vi "ConfigUtilities - Get Tx Packet Information.vi"(8 "error in (no error)":errorcluster, 11 "Custom Device Ref in":T1 format="%.0x") -> (0 "error out":errorcluster, 1 "Tx Ref Array":T2(array[cluster]) {"VS Refs" format="%.0x"}, 2 "Tx Packet Info Array":T3[](array[typedef]) {"Endianness" items=["big-endian"=0, "little-indian"=2]}, 3 "Custom Device Ref out":T1 format="%.0x")   [LabVIEW 2016, in "UDP-Custom-Device System Explorer.lvlib"]
uses:
  UDP-Custom-Device System Explorer.lvlib
  Shared/Tx.PacketInfo.ctl
  Types/Channel Data Type.ctl
  Shared/Header Details.ctl
  <vilib>/NI Veristand/Custom Device API/Custom Device Item Ref.ctl
  Shared/Constants.vi
  <vilib>/NI Veristand/Custom Device API/Get Item Property (I32).vi
  <vilib>/NI Veristand/Custom Device API/Get Item Property (String).vi
  <vilib>/NI Veristand/Custom Device API/Get Item Property (U16).vi
  <vilib>/NI Veristand/Custom Device API/Get Item Property (Boolean).vi
  <vilib>/NI Veristand/Custom Device API/Get Item Property (U32).vi
  Shared/UDP-Custom-Device Shared.lvlib
  <vilib>/NI VeriStand/Custom Device API/Custom Device API.lvlib
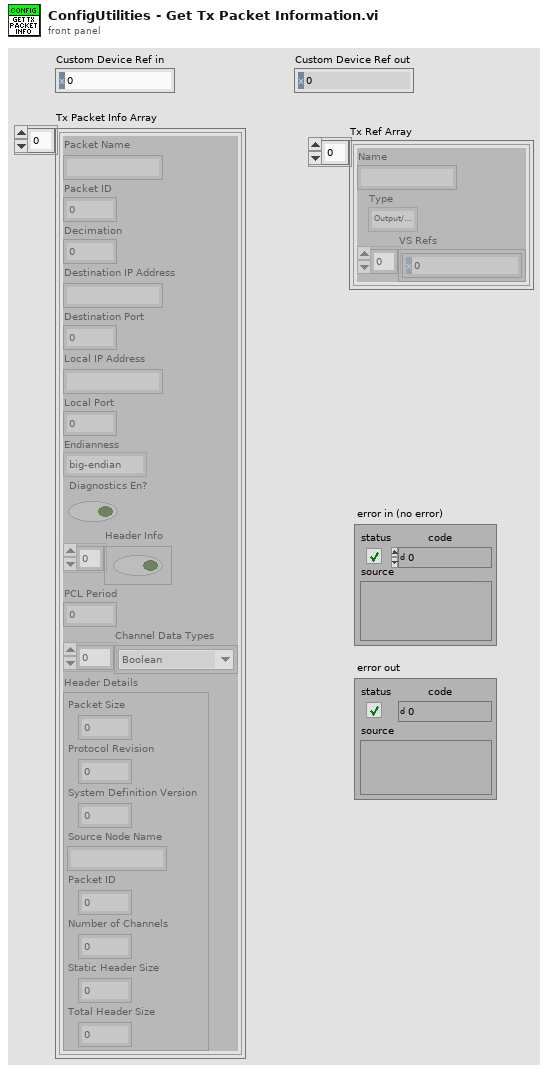
[diagram p1: front panel]
types:
  T1 = typedef "Custom Device API.lvlib/Custom Device Item Ref.ctl" = u64
  T2 = cluster{"Name":string, "Type":enum16{"Output/Write", "Input/Read", "Input/ReadWrite"}, "VS Refs":T1[]}[]
  T3 = typedef "UDP-Custom-Device Shared.lvlib/Tx.PacketInfo.ctl" = cluster{"Packet Name":string, "Packet ID":i32, "Decimation":u16, "Destination IP Address":string, "Destination Port":i32, "Local IP Address":string, "Local Port":i32, "Endianness":u16, "Diagnostics En?":bool, "Header Info":bool[], "PCL Period":u32, "Channel Data Types":T4[], "Header Details":T5}
  T4 = typedef "UDP-Custom-Device Shared.lvlib/Channel Data Type.ctl" = enum16{"Boolean", "Single", "Double", "I8", "I16", "I32", "I64", "U8", "U16", "U32", "U64"}
  T5 = typedef "UDP-Custom-Device Shared.lvlib/Header Details.ctl" = cluster{"Packet Size":u16, "Protocol Revision":u8, "System Definition Version":u64, "Source Node Name":string, "Packet ID":u32, "Number of Channels":u32, "Static Header Size":u16, "Total Header Size":u16}
  T6 = cluster{"Name":string, "Type":enum16{"Output/Write", "Input/Read", "Input/ReadWrite"}, "VS Refs":T1[]}
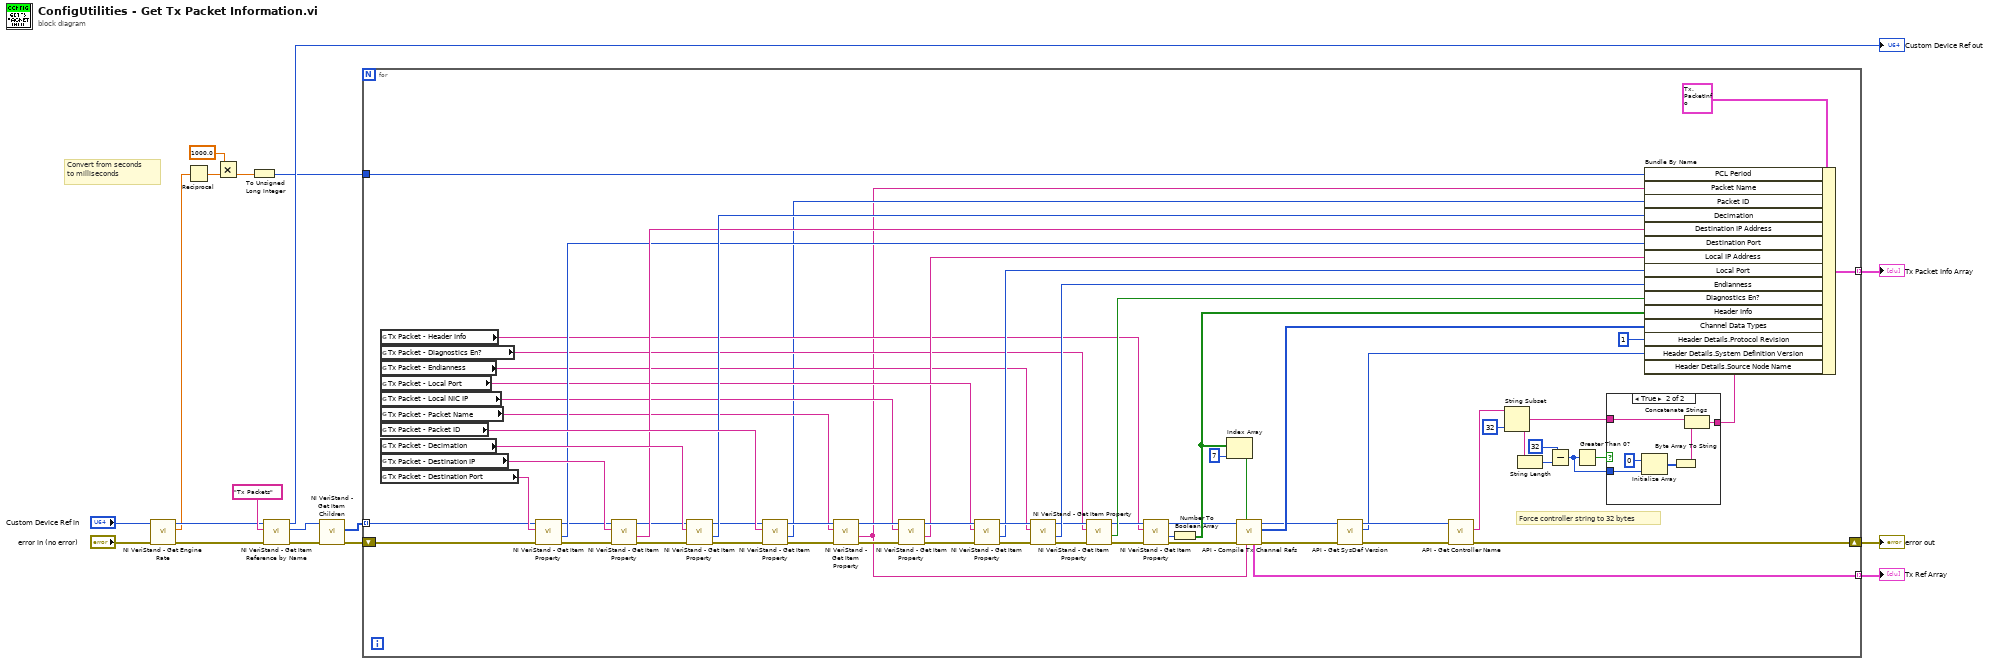
[diagram p0: block diagram]
diagram:
  # "Convert from seconds\nto milliseconds"
  n1 = call <vilib>:"NI VeriStand - Get Engine Rate.vi"("error in (no error)"="error in (no error)", "Item Ref in"="Custom Device Ref in") -> ("error out"=w7:errorcluster, "Rate (Hz)"=w5:dbl, "Item Ref out"=w6:T1)  [unwired: 7 in]
  n2 = Reciprocal(x=w5) -> (1/x=w1:dbl)
  n3 = Multiply(x=1000.0, y=w1) -> (x*y=w3:dbl)
  n4 = To Unsigned Long Integer(number=w3) -> (unsigned 32bit integer=w4:u32)
  n5 = call <vilib>:"NI VeriStand - Get Item Reference by Name.vi"("error in (no error)"=w7, "Item Name"="Tx Packets", "Parent Ref in"=w6) -> ("error out"=w13:errorcluster, "Item Ref"=w11:T1, "Parent Ref out"=→"Custom Device Ref out":T1)  [unwired: 5 in, 1 out]
  n6 = call <vilib>:"NI VeriStand - Get Item Children.vi"("error in (no error)"=w13, "Item Ref in"=w11) -> ("error out"=w16:errorcluster, "Child Refs"=w15:T1[])  [unwired: 6 in, 2 out]
  n7 = for {
    shift-right: [w32] -> w18
    shift-left: w16 -> [w83]
    tunnel: [w66] -> w17 mode=indexing
    tunnel: w15 -> [w65] mode=indexing
    tunnel: [w35] -> w14 mode=indexing
    tunnel: w4 -> [w44]
    # "Force controller string to 32 bytes"
    n8 = global read "Constants.vi" "Tx Packet - Header Info"() -> (w46:string)
    n9 = global read "Constants.vi" "Tx Packet - Diagnostics En?"() -> (w48:string)
    n10 = global read "Constants.vi" "Tx Packet - Endianness"() -> (w52:string)
    n11 = global read "Constants.vi" "Tx Packet - Local Port"() -> (w59:string)
    n12 = global read "Constants.vi" "Tx Packet - Local NIC IP"() -> (w60:string)
    n13 = global read "Constants.vi" "Tx Packet - Packet Name"() -> (w43:string)
    n14 = global read "Constants.vi" "Tx Packet - Packet ID"() -> (w79:string)
    n15 = global read "Constants.vi" "Tx Packet - Decimation"() -> (w80:string)
    n16 = global read "Constants.vi" "Tx Packet - Destination IP"() -> (w81:string)
    n17 = global read "Constants.vi" "Tx Packet - Destination Port"() -> (w82:string)
    n18 = call-poly <vilib>:"NI VeriStand - Get Item Property.vi"("error in (no error)"=w83, "Property Name"=w82, "Item Ref in"=w65) -> ("error out"=w71:errorcluster, "Value"=w76:i32, "Item Ref out"=w75:T1)  [unwired: 5 in, 1 out]
    n19 = call-poly <vilib>:"NI VeriStand - Get Item Property.vi"("error in (no error)"=w71, "Property Name"=w81, "Item Ref in"=w75) -> ("error out"=w70:errorcluster, "Value"=w77:string, "Item Ref out"=w74:T1)  [unwired: 5 in, 1 out]
    n20 = call-poly <vilib>:"NI VeriStand - Get Item Property.vi"("error in (no error)"=w70, "Property Name"=w80, "Item Ref in"=w74) -> ("error out"=w69:errorcluster, "Value"=w78:u16, "Item Ref out"=w73:T1)  [unwired: 5 in, 1 out]
    n21 = call-poly <vilib>:"NI VeriStand - Get Item Property.vi"("error in (no error)"=w69, "Property Name"=w79, "Item Ref in"=w73) -> ("error out"=w68:errorcluster, "Value"=w40:i32, "Item Ref out"=w72:T1)  [unwired: 5 in, 1 out]
    n22 = call-poly <vilib>:"NI VeriStand - Get Item Property.vi"("error in (no error)"=w68, "Property Name"=w43, "Item Ref in"=w72) -> ("error out"=w64:errorcluster, "Value"=w36:string, "Item Ref out"=w63:T1)  [unwired: 5 in, 1 out]
    n23 = call-poly <vilib>:"NI VeriStand - Get Item Property.vi"("error in (no error)"=w64, "Property Name"=w60, "Item Ref in"=w63) -> ("error out"=w61:errorcluster, "Value"=w55:string, "Item Ref out"=w62:T1)  [unwired: 5 in, 1 out]
    n24 = call-poly <vilib>:"NI VeriStand - Get Item Property.vi"("error in (no error)"=w61, "Property Name"=w59, "Item Ref in"=w62) -> ("error out"=w57:errorcluster, "Value"=w54:i32, "Item Ref out"=w58:T1)  [unwired: 5 in, 1 out]
    n25 = call-poly <vilib>:"NI VeriStand - Get Item Property.vi"("error in (no error)"=w57, "Property Name"=w52, "Item Ref in"=w58) -> ("error out"=w56:errorcluster, "Value"=w53:u16, "Item Ref out"=w50:T1)  [unwired: 5 in, 1 out]
    n26 = call-poly <vilib>:"NI VeriStand - Get Item Property.vi"("error in (no error)"=w56, "Property Name"=w48, "Item Ref in"=w50) -> ("error out"=w51:errorcluster, "Value"=w49:bool, "Item Ref out"=w47:T1)  [unwired: 5 in, 1 out]
    n27 = call-poly <vilib>:"NI VeriStand - Get Item Property.vi"("error in (no error)"=w51, "Property Name"=w46, "Item Ref in"=w47) -> ("error out"=w42:errorcluster, "Value"=w45:u32, "Item Ref out"=w34:T1)  [unwired: 5 in, 1 out]
    n28 = Number To Boolean Array(number=w45) -> (Boolean array=w39:bool[])
    n29 = Index Array(array=w39, index=7) -> (element=w37:bool)
    n30 = call "API - Compile Tx Channel Refs.vi"("Packet Name"=w36, "Timestamp Present?"=w37, "error in (no error)"=w42, "Item Ref in"=w34) -> ("error out"=w21:errorcluster, "Data types"=w33:T4[], "Item Ref out"=w23:T1, "Tx Ref Array"=w35:T6)  [unwired: 4 in]
    n31 = call "API - Get SysDef Version.vi"("error in (no error)"=w21, "Packet Ref In"=w23) -> ("error out"=w20:errorcluster, "Encoded Version"=w19:u64, "Packet Ref out"=w22:T1)  [unwired: 6 in, 1 out]
    n32 = call "API - Get Controller Name.vi"("error in (no error)"=w20, "Packet Ref In"=w22) -> ("error out"=w32:errorcluster, "Name"=w31:string)  [unwired: 7 in, 1 out]
    n33 = String Subset(string=w31, length (rest)=32 ("length (rest)")) -> (substring=w25:string)  [unwired: 1 in]
    n34 = String Length(string=w25) -> (length=w28:i32)
    n35 = Subtract(x=32 ("length (rest)"), y=w28) -> (x-y=w26:i32)
    n36 = Greater Than 0?(x=w26) -> (x > 0?=w27:bool)
    n37 = case shown="True" w27 {
      tunnel: w26 -> [_ w90]
      tunnel: w25 -> [w84 w87]
      tunnel: [w84 w85] -> w24
      frame False {
      }
      frame True {
        n38 = Initialize Array(u8 0, w90) -> (w88:u8[])
        n39 = Byte Array To String(unsigned byte array=w88) -> (string=w86:string)
        n40 = Concatenate Strings(w87, w86) -> (w85:string)
      }
    }
    n41 = Bundle By Name(cluster=T3 {"Packet Name"="", "Packet ID"=0, "Decimation"=0, "Destination IP Address"="", "Destination Port"=0, "Local IP Address"="", "Local Port"=0, "Endianness"=0, "Diagnostics En?"=FALSE, "Header Info"=[], "PCL Period"=0, "Channel Data Types"=[], "Header Details"={"Packet Size"=0, "Protocol Revision"=0, "System Definition Version"=0, "Source Node Name"="", "Packet ID"=0, "Number of Channels"=0, "Static Header Size"=0, "Total Header Size"=0}} ("Packet Info"), "PCL Period"=w44, "Packet Name"=w36, "Packet ID"=w40, "Decimation"=w78, "Destination IP Address"=w77, "Destination Port"=w76, "Local IP Address"=w55, "Local Port"=w54, "Endianness"=w53, "Diagnostics En?"=w49, "Header Info"=w39, "Channel Data Types"=w33, "Header Details.Protocol Revision"=u8 1, "Header Details.System Definition Version"=w19, "Header Details.Source Node Name"=w24) -> (w66:T3)
  }
  "Tx Packet Info Array" <- w17
  "error out" <- w18
  "Tx Ref Array" <- w14
